vi "WriteSectionFrame.vi"(8 "section name":string, 9 "section index":i32, 10 "section frame":i32, 11 "[base]\\traces\\[expname]_sections.txt":path) -> ()   [LabVIEW 2011]
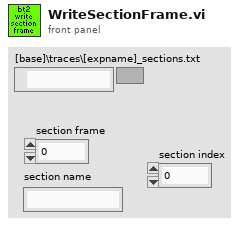
[diagram p1: front panel]
types:
  T1 = enum16{"open", "replace", "create", "open or create", "replace or create", "replace or create with confirmation"}
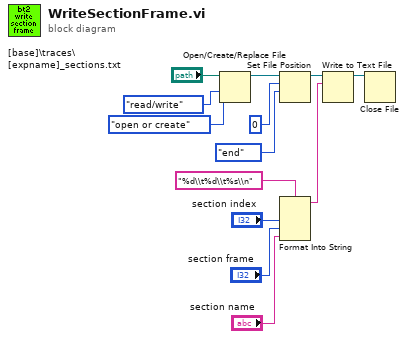
[diagram p0: block diagram]
diagram:
  n1 = Open/Create/Replace File(file path (use dialog)="[base]\\traces\\[expname]_sections.txt", operation (0:open)=T1."open or create", access (0:read/write)=enum16{"read/write", "read-only", "write-only"}."read/write") -> (refnum out=w2:refnum<file>)  [unwired: 3 in, 2 out]
  n2 = Set File Position(offset (in bytes) (0)=i64 0, refnum=w2, from (0:start)=enum16{"start", "end", "current"}."end") -> (refnum out=w11:refnum<file>)  [unwired: 1 in, 1 out]
  n3 = Format Into String(format string="%d\\t%d\\t%s\\n", "section index", "section frame", "section name") -> (resulting string=w7:string)  [unwired: 2 in, 1 out]
  n4 = Write to Text File(file (use dialog)=w11, text=w7) -> (refnum out=w6:refnum<file>)  [unwired: 2 in, 2 out]
  n5 = Close File(refnum=w6) -> ()  [unwired: 1 in, 2 out]
